vi "inspect lv recurse type names.vi"(8 "error in (no error)":errorcluster, 11 "ProjectItem in":refnum<vi>) -> (0 "error out":errorcluster, 2 "Type String":string[](array[string]), 3 "ProjectItem out":refnum<vi>)   [LabVIEW 2023]
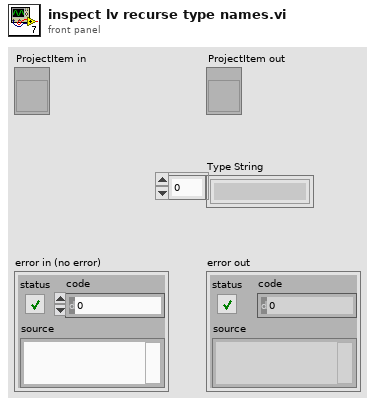
[diagram p1: front panel]
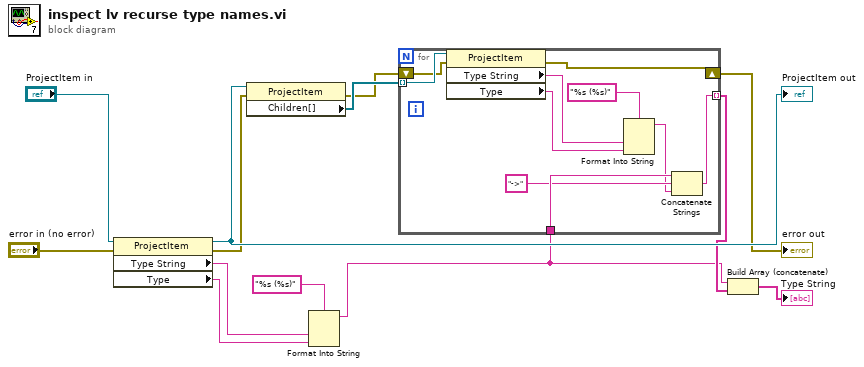
[diagram p0: block diagram]
diagram:
  n1 = property class="ProjectItem"(reference="ProjectItem in", error in="error in (no error)") -> (reference out=w11:refnum<vi>, error out=w6:errorcluster, "Type String"=w2:string, "Type"=w3:string)
  "ProjectItem out" <- w11
  n2 = property class="ProjectItem"(reference=w11, error in=w6) -> (error out=w7:errorcluster, "Children[]"=w10:refnum<vi>[])  [unwired: 1 out]
  n3 = Format Into String(format string="%s (%s)", w2, w3) -> (resulting string=w1:string)  [unwired: 2 in, 1 out]
  n4 = for {
    tunnel: w10 -> [w23] mode=indexing
    tunnel: w1 -> [w22]
    tunnel: [w20] -> w9 mode=indexing
    shift-right: [w18] -> w5
    shift-left: w7 -> [w19]
    n5 = property class="ProjectItem"(reference=w23, error in=w19) -> (error out=w18:errorcluster, "Type String"=w15:string, "Type"=w14:string)  [unwired: 1 out]
    n6 = Format Into String(format string="%s (%s)", w15, w14) -> (resulting string=w16:string)  [unwired: 2 in, 1 out]
    n7 = Concatenate Strings(w22, "->" ("string"), w16) -> (w20:string)
  }
  "error out" <- w5
  n8 = Build Array (concatenate)(w1, w9) -> (→"Type String":string[])
